vi "ABB Norma 5000 Averaging Status.vi"(8 "error in (no error)":errorcluster, 10 "Timeout":dbl format="%.2f", 11 "VISA session":refnum<visa-resource-name>) -> (0 "error out":errorcluster, 2 "State":i32(ring) items=["In Progress", "Complete"], 3 "dup VISA session":refnum<visa-resource-name>)   [LabVIEW 2017]
doc: "This VI queries the averaging status synchronously or asynchronously. In synchronous mode this VI waits for the averaging to complete."
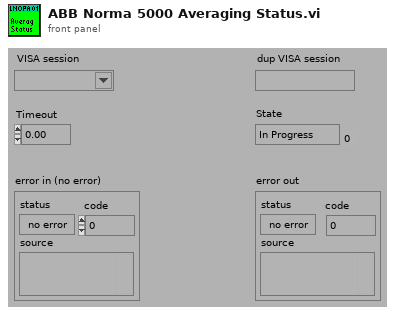
[diagram p1: front panel]
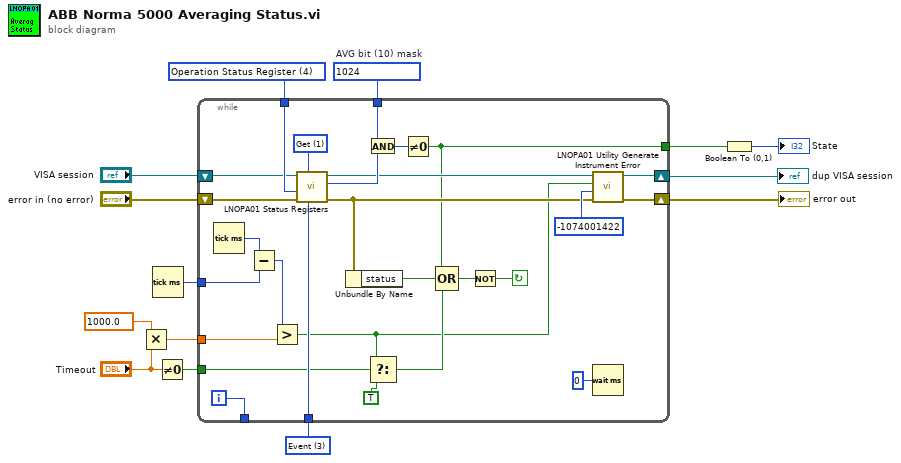
[diagram p0: block diagram]
diagram:
  w12 = u16 1024  # AVG bit (10) mask
  w13 = 3 items=["Condition", "Positive Transition", "Negative Transition", "Event", "Enable"] ("Register Part")
  w14 = 4 items=["Status Byte (STB)", "Service Request Enable Register (SRE)", "Standard Event Status Register (ESR)", "Standard Event Status Enable Register (ESE)", "Operation Status Register", "Questionable Status Register", "Questionable Voltage Status Register", "Questionable Current Status Register"] ("Register")
  n1 = Multiply(x=1000.0 ("y"), y="Timeout") -> (x*y=w9:dbl)
  n2 = Tick Count (ms)() -> (millisecond timer value=w10:u32)
  n3 = Not Equal To 0?(x="Timeout") -> (x != 0?=w1:bool)
  n4 = while {
    tunnel: [w16] -> _
    tunnel: w1 -> [w20]
    shift-left: "VISA session" -> [w31]
    shift-right: [w24] -> w5
    shift-left: "error in (no error)" -> [w32]
    shift-right: [w30] -> w6
    tunnel: w9 -> [w35]
    tunnel: w10 -> [w28]
    tunnel: [w21] -> w4
    tunnel: w12 -> [w38]
    tunnel: w13 -> [w40]
    tunnel: w14 -> [w41]
    i -> [w16]
    stop <- w22 continue-if-true
    w33 = 1 items=["Set", "Get"] ("Operation (0:Set)")
    n5 = Tick Count (ms)() -> (millisecond timer value=w29:u32)
    n6 = Subtract(x=w29, y=w28) -> (x-y=w36:u32)
    n7 = Greater?(x=w36, y=w35) -> (0:w17:bool)
    n8 = call "LNOPA01 Status Registers.vi"("Register Part"=w40, "Operation"=w33, "error in (no error)"=w32, "Register"=w41, "VISA session"=w31) -> ("error out"=w26:errorcluster, "State"=w39:u16, "dup VISA session"=w25:refnum<visa-resource-name>)  [unwired: 4 in]
    n9 = Unbundle By Name(w26) -> ("status"=w23:bool)
    n10 = And(x=w38, y=w39) -> (x .and. y?=w37:u16)
    n11 = Select(t=w17, s=w20, f=TRUE) -> (s? t:f=w18:bool)
    n12 = Not Equal To 0?(x=w37) -> (x != 0?=w21:bool)
    n13 = Compound Arithmetic op=OR(w21, w23, w18) -> (w34:bool)
    n14 = Not(x=w34) -> (.not. x?=w22:bool)
    n15 = call "LNOPA01 Utility Generate Instrument Error.vi"("error in"=w26, "Code"=-1074001422, "Status"=w17, "VISA session"=w25) -> ("error out"=w30:errorcluster, "dup VISA session"=w24:refnum<visa-resource-name>)  [unwired: 6 in]
    n16 = Wait (ms)(milliseconds to wait=u32 0) -> ()  [unwired: 1 out]
  }
  "error out" <- w6
  "dup VISA session" <- w5
  n17 = Boolean To (0,1)(Boolean=w4) -> (0, 1=→"State":i16)
